vi "monitor_v2.vi"() -> ()   [LabVIEW 2024]
panel:
  in  "load":dbl(slide) scale=40.0..120.0
  in  "swing":dbl(slide) scale=0.0..180.0
  in  "boom":dbl(slide) scale=40.0..80.0
  out "Waveform Chart 2":T1(graph)
  out "Waveform Chart":dbl(graph)
  in  "stop":bool
  out "return value":dbl[](array[numeric])
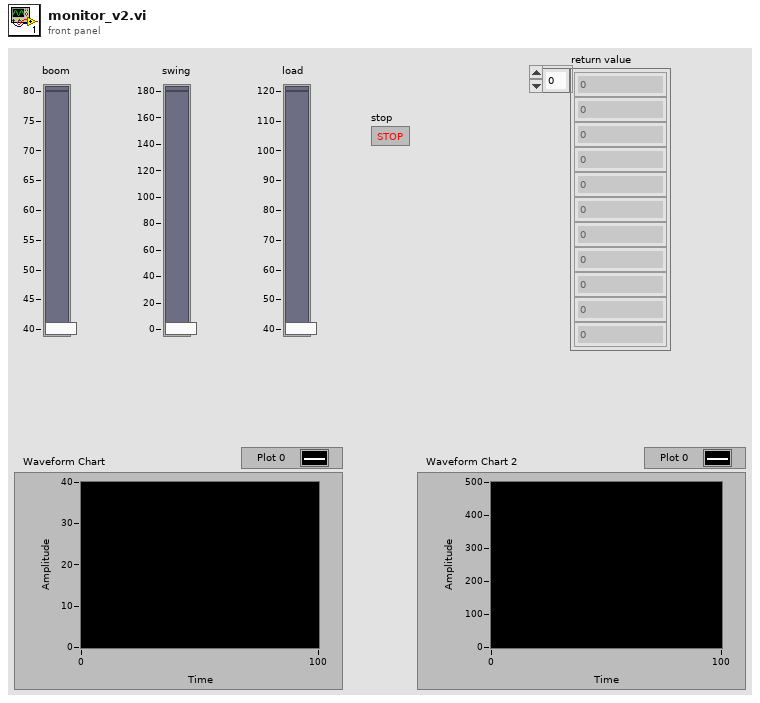
[diagram p1: front panel]
types:
  T1 = cluster{"[0]":dbl, "[1]":dbl, "[2]":dbl, "[3]":dbl, "[4]":dbl, "[5]":dbl, "[6]":dbl, "[7]":dbl, "[8]":dbl}
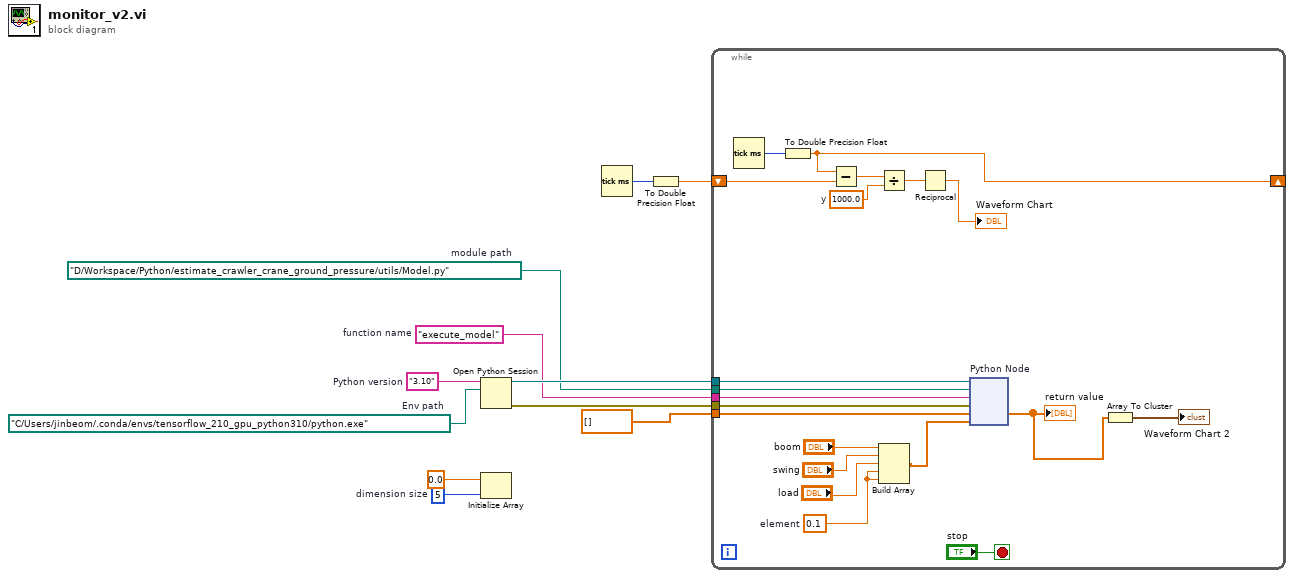
[diagram p0: block diagram]
diagram:
  w4 = 5  # dimension size
  w6 = "execute_model"  # function name
  w7 = path "D:/Workspace/Python/estimate_crawler_crane_ground_pressure/utils/Model.py"  # module path
  w11 = path "C:/Users/jinbeom/.conda/envs/tensorflow_210_gpu_python310/python.exe"  # Env path
  w10 = "3.10"  # Python version
  n1 = Open Python Session(python version=w10, python path=w11) -> (session out=w9:refnum<k35>, error out=w8:errorcluster)  [unwired: 1 in]
  n2 = Initialize Array "Initialize Array"(0.0, w4) -> ()  [unwired: 1 out]
  n3 = Tick Count (ms)() -> (millisecond timer value=w3:u32)
  n4 = To Double Precision Float(number=w3) -> (double precision float=w2:dbl)
  n5 = while {
    tunnel: w9 -> [w31]
    tunnel: w8 -> [w30]
    tunnel: w7 -> [w29]
    tunnel: w6 -> [w28]
    shift-right: [w25] -> _
    shift-left: w2 -> [w24]
    tunnel: dbl[] [] -> [w17]
    stop <- "stop" stop-if-true
    w13 = 0.1  # element
    w22 = 1000.0  # y
    n6 = Tick Count (ms)() -> (millisecond timer value=w26:u32)
    n7 = To Double Precision Float(number=w26) -> (double precision float=w25:dbl)
    n8 = Subtract(x=w25, y=w24) -> (x-y=w23:dbl)
    n9 = Divide(x=w23, y=w22) -> (x/y=w21:dbl)
    n10 = Build Array("boom", "swing", "load", w13, w13) -> (w12:dbl[])
    n11 = Reciprocal(x=w21) -> (1/x=→"Waveform Chart":dbl)
    n12 = node "Python Node"(w31, w29, w28, w30, w17, w12) -> (w19:dbl[])  [unwired: 1 in, 4 out]
    "return value" <- w19
    n13 = Array To Cluster(array=w19) -> (cluster=→"Waveform Chart 2":T1)
  }
